vi "从板信息配置.vi"(2 "从板信息查看":string[][](table)) -> (0 "输出数组":string[][](array[string]), 1 "布尔":bool)   [LabVIEW 2013]
panel:
  in  "自动计算通道电压":bool
  in  "通道电压清零":bool
  in  "保险位置清零":bool
  in  "停止":bool
  in  "整车CAN测试":bool
  in  "保险位置":bool[][](array[boolean])
  in  "从板信息":string[][](table)=[["电压个数", "", "温度个数", "", "主板温度个数", "", "主板温度起始值"], ["电压起始值", "", "温度起始值", "", "从板1温度个数", "", "从板1主板温度起始值"]]
  in  "20个通道电压个数":u8[](array[numeric]) max=12
  # "1"
  # "2"
  # "3"
  # "4"
  # "5"
  # "6"
  # "7"
  # "8"
  # "9"
  # "10"
  # "11"
  # "12"
  # "第一通道"
  # "第二通道"
  # "第三通道"
  # "第四通道"
  # "第五通道"
  # "第六通道"
  # "第七通道"
  # "第八通道"
  # "第九通道"
  # "第十通道"
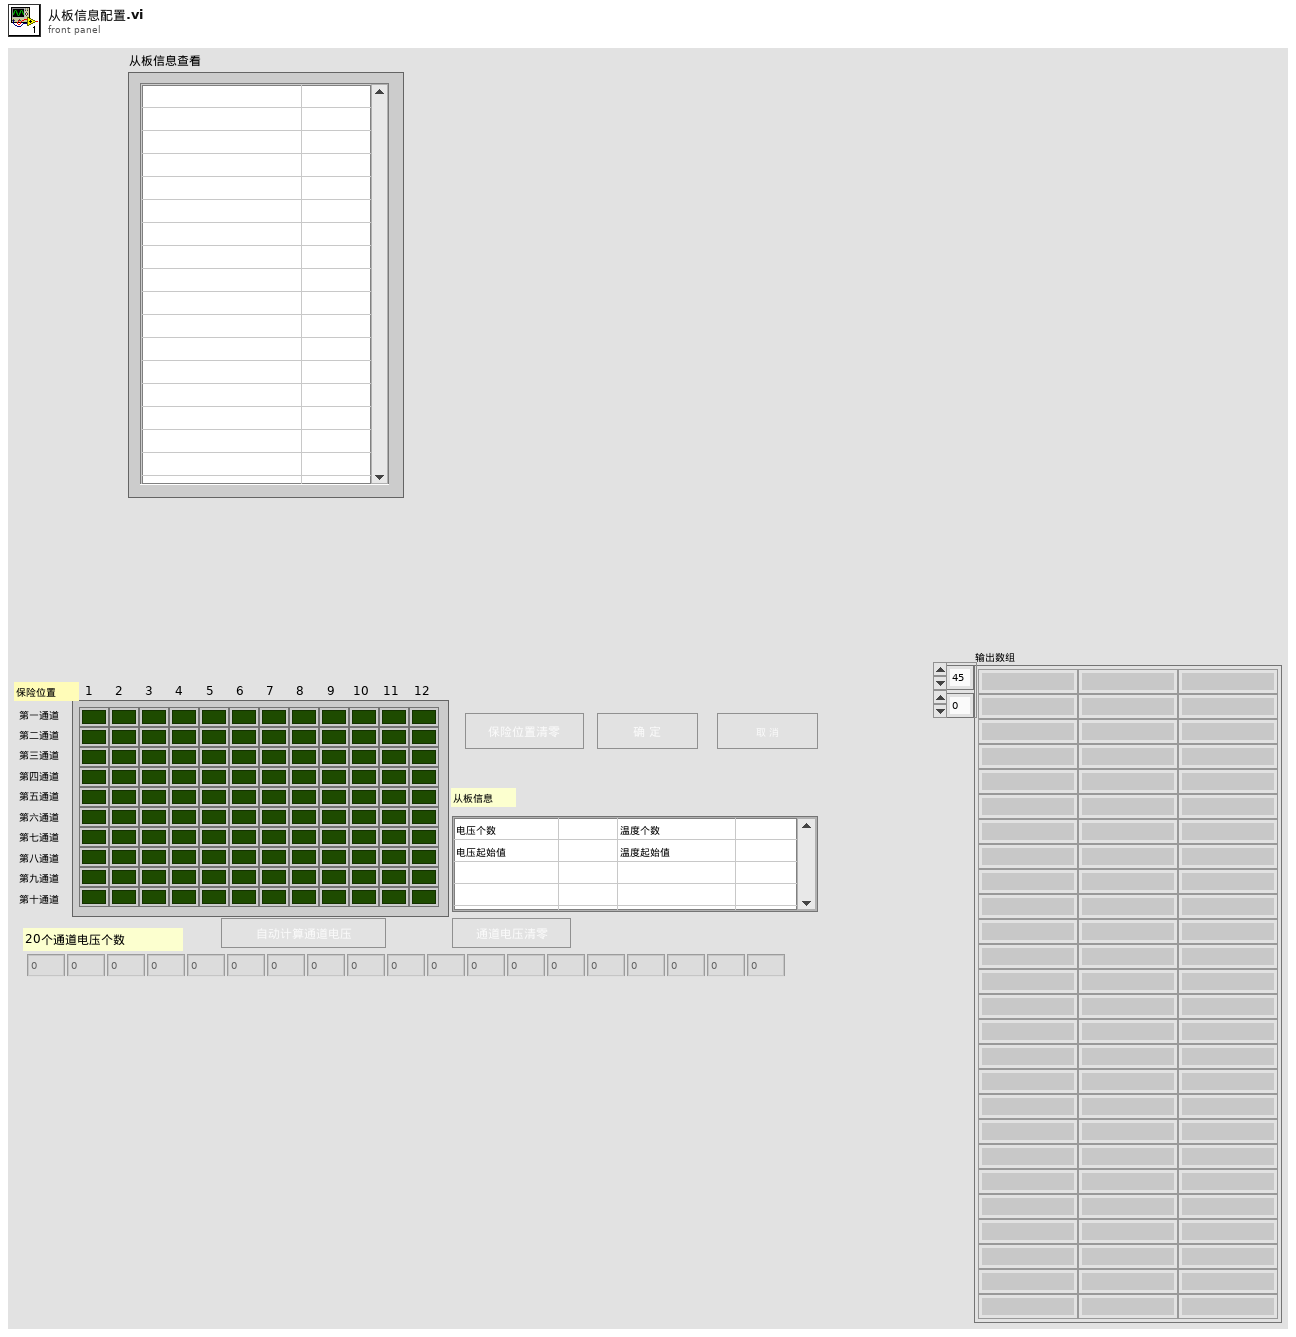
[diagram p1: front panel]
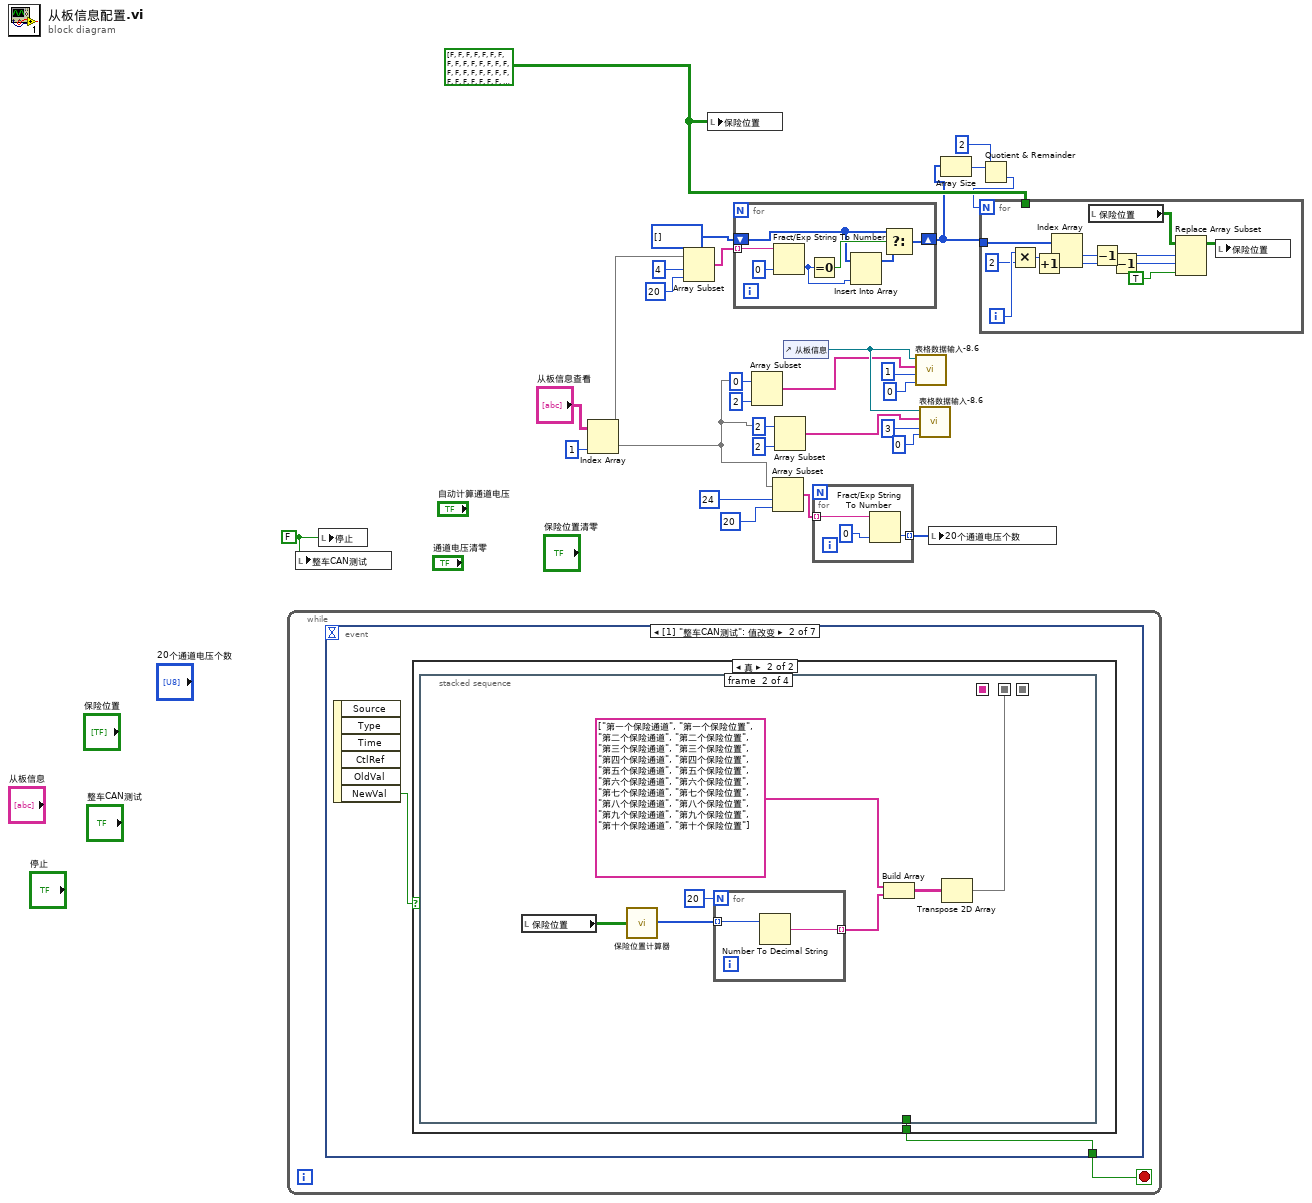
[diagram p0: block diagram]
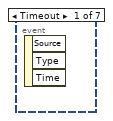
[diagram p2: hidden frame]
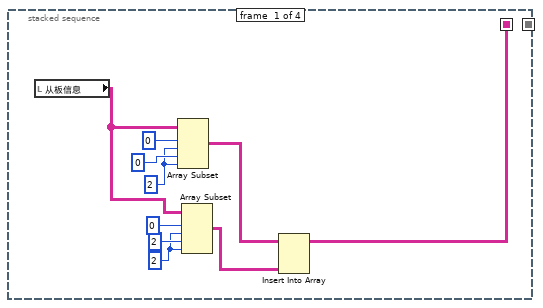
[diagram p4: hidden frame]
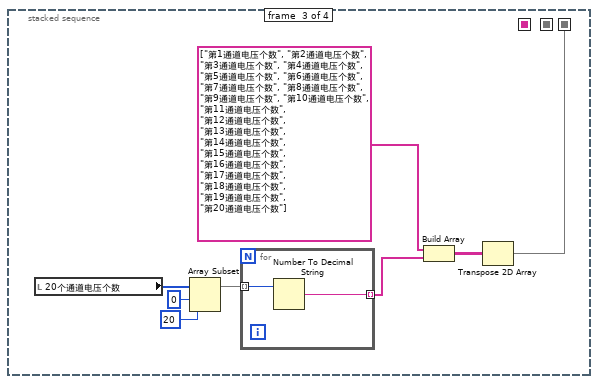
[diagram p5: hidden frame]
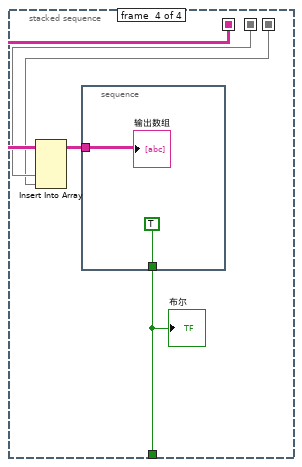
[diagram p6: hidden frame]
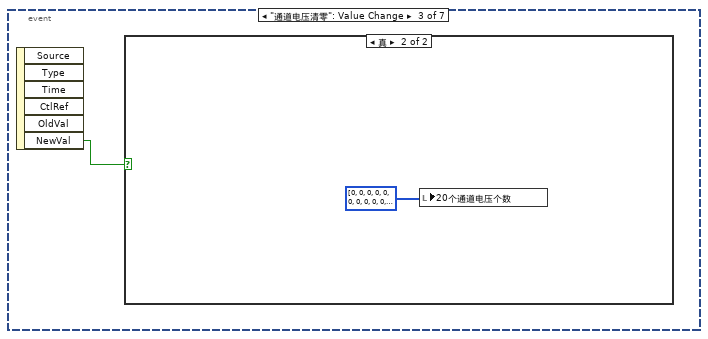
[diagram p7: hidden frame]
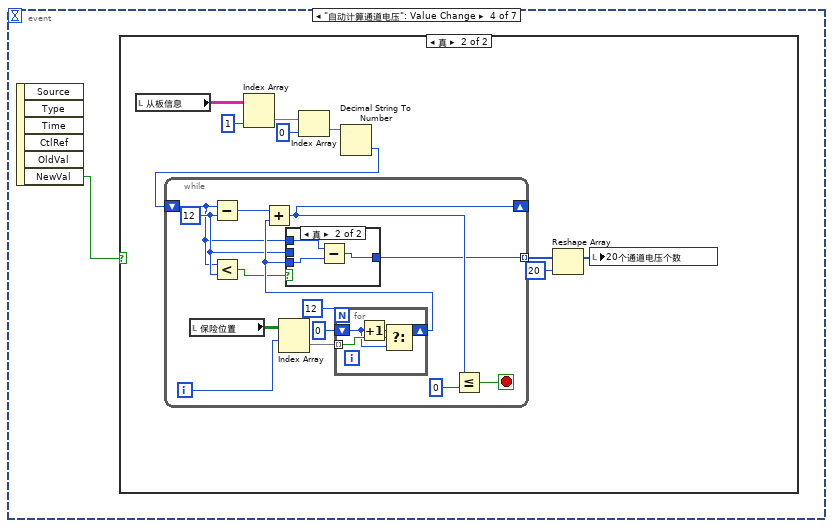
[diagram p9: hidden frame]
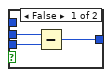
[diagram p11: hidden frame]
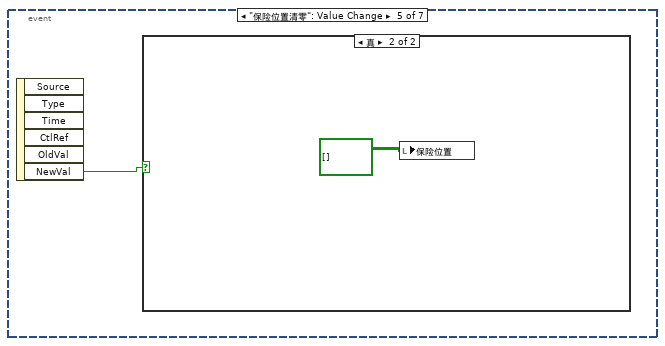
[diagram p12: hidden frame]
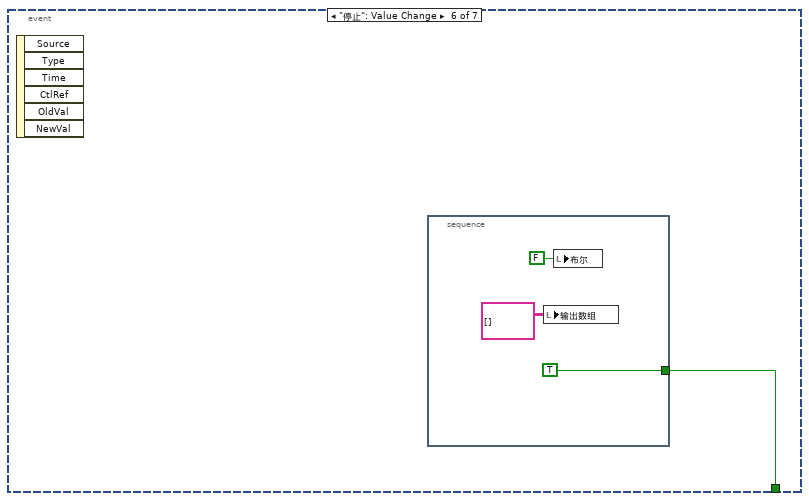
[diagram p14: hidden frame]
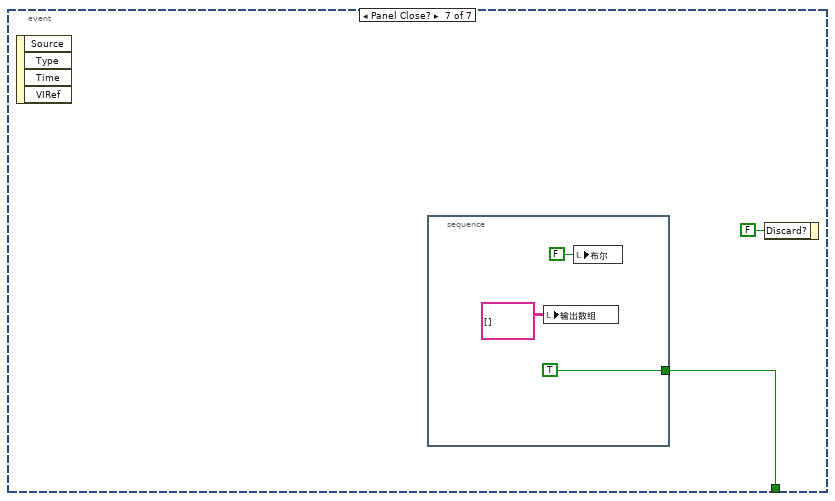
[diagram p15: hidden frame]
diagram:
  w6 = bool[][] [[FALSE, FALSE, FALSE, FALSE, FALSE, FALSE, FALSE, FALSE, FALSE, FALSE, FALSE, FALSE], [FALSE, FALSE, FALSE, FALSE, FALSE, FALSE, FALSE, FALSE, FALSE, FALSE, FALSE, FALSE], [FALSE, FALSE, FALSE, FALSE, FALSE, FALSE, FALSE, FALSE, FALSE, FALSE, FALSE, FALSE], [FALSE, FALSE, FALSE, FALSE, FALSE, FALSE, FALSE, FALSE, FALSE, FALSE, FALSE, FALSE], [FALSE, FALSE, FALSE, FALSE, FALSE, FALSE, FALSE, FALSE, FALSE, FALSE, FALSE, FALSE], [FALSE, FALSE, FALSE, FALSE, FALSE, FALSE, FALSE, FALSE, FALSE, FALSE, FALSE, FALSE], [FALSE, FALSE, FALSE, FALSE, FALSE, FALSE, FALSE, FALSE, FALSE, FALSE, FALSE, FALSE], [FALSE, FALSE, FALSE, FALSE, FALSE, FALSE, FALSE, FALSE, FALSE, FALSE, FALSE, FALSE], [FALSE, FALSE, FALSE, FALSE, FALSE, FALSE, FALSE, FALSE, FALSE, FALSE, FALSE, FALSE], [FALSE, FALSE, FALSE, FALSE, FALSE, FALSE, FALSE, FALSE, FALSE, FALSE, FALSE, FALSE]]
  w28 = FALSE ("取消按钮")
  n1 = while {
    stop <- w29 stop-if-true
    n2 = event shown="[1] \"整车CAN测试\": 值改变" {
      selector: _ -> [_ _ _ _ _ _ _]
      dyn-events: _ -> [_ _ _ _ _ _ _]
      timeout: _ -> [_ _ _ _ _ _ _]
      tunnel: [_ w30 _ _ _ w107 w112] -> w29
      event Timeout {
        n3 = event-data() -> ()  [unwired: 1 in, 3 out]
      }
      event "整车CAN测试": Value Change {
        n4 = event-data() -> ("NewVal"=w31:bool)  [unwired: 1 in, 5 out]
        n5 = case shown="真" w31 {
          tunnel: [_ w32] -> w30
          frame False {
          }
          frame True {
            n6 = stacked-sequence {
              seq-local: [w35 _ _ _] -> [_ _ _ w64]
              seq-local: [_ w44 _ _] -> [_ _ _ w63]
              seq-local: [_ _ w55 _] -> [_ _ _ w62]
              tunnel: [_ _ _ w65] -> w32
              frame #0 {
                w33 = 2 ("索引")
                w34 = 2 ("索引")
                n7 = local read "从板信息"() -> (w38:string[][])
                n8 = Array Subset(array=w38, index (row)=0 ("索引"), length (row)=w34, index (col)=0 ("索引"), length (col)=w34) -> (w37:string[][])
                n9 = Array Subset(array=w38, index (row)=0 ("索引"), length (row)=w33, index (col)=2 ("索引"), length (col)=w33) -> (w36:string[][])
                n10 = Insert Into Array(array=w37, new element=w36) -> (w35:string[][])  [unwired: 2 in]
              }
              frame #1 {
                n11 = local read "保险位置"() -> (w49:bool[][])
                n12 = call "保险位置计算器.vi"("保险位置"=w49) -> ("输出数组"=w48:i32[])
                n13 = for {
                  N: 20 -> [_]
                  tunnel: w48 -> [w51] mode=indexing
                  tunnel: [w50] -> w47 mode=indexing
                  n14 = Number To Decimal String(number=w51) -> (decimal integer string=w50:string)  [unwired: 1 in]
                }
                n15 = Build Array(string[] ["第一个保险通道", "第一个保险位置", "第二个保险通道", "第二个保险位置", "第三个保险通道", "第三个保险位置", "第四个保险通道", "第四个保险位置", "第五个保险通道", "第五个保险位置", "第六个保险通道", "第六个保险位置", "第七个保险通道", "第七个保险位置", "第八个保险通道", "第八个保险位置", "第九个保险通道", "第九个保险位置", "第十个保险通道", "第十个保险位置"], w47) -> (w45:string[][])
                n16 = Transpose 2D Array(2D array=w45) -> (transposed array=w44:string[][])
              }
              frame #2 {
                n17 = local read "20个通道电压个数"() -> (w59:u8[])
                n18 = Array Subset(array=w59, index=0 ("索引"), length=20 ("长度")) -> (w54:u8[])
                n19 = for {
                  tunnel: w54 -> [w61] mode=indexing
                  tunnel: [w60] -> w58 mode=indexing
                  n20 = Number To Decimal String(number=w61) -> (decimal integer string=w60:string)  [unwired: 1 in]
                }
                n21 = Build Array(string[] ["第1通道电压个数", "第2通道电压个数", "第3通道电压个数", "第4通道电压个数", "第5通道电压个数", "第6通道电压个数", "第7通道电压个数", "第8通道电压个数", "第9通道电压个数", "第10通道电压个数", "第11通道电压个数", "第12通道电压个数", "第13通道电压个数", "第14通道电压个数", "第15通道电压个数", "第16通道电压个数", "第17通道电压个数", "第18通道电压个数", "第19通道电压个数", "第20通道电压个数"], w58) -> (w56:string[][])
                n22 = Transpose 2D Array(2D array=w56) -> (transposed array=w55:string[][])
              }
              frame #3 {
                n23 = Insert Into Array(array=w64, new element #1=w63, new element #2=w62) -> (w66:string[][])  [unwired: 2 in]
                n24 = stacked-sequence {
                  tunnel: w66 -> [w68]
                  tunnel: [TRUE] -> w65
                  frame #0 {
                    "输出数组" <- w68
                  }
                }
                "布尔" <- w65
              }
            }
          }
        }
      }
      event "通道电压清零": Value Change {
        n25 = event-data() -> ("NewVal"=w69:bool)  [unwired: 1 in, 5 out]
        n26 = case shown="真" w69 {
          frame False {
          }
          frame True {
            n27 = local write "20个通道电压个数"(i32[] [0, 0, 0, 0, 0, 0, 0, 0, 0, 0, 0, 0, 0, 0, 0, 0, 0, 0, 0, 0, 0] ("20个通道电压个数")) -> ()
          }
        }
      }
      event "自动计算通道电压": Value Change {
        n28 = event-data() -> ("NewVal"=w71:bool)  [unwired: 1 in, 5 out]
        n29 = case shown="真" w71 {
          frame False {
          }
          frame True {
            n30 = local read "从板信息"() -> (w80:string[][])
            n31 = Index Array(array=w80, index (col)=1 ("禁用的索引 (列)")) -> (element=w78:string[])  [unwired: 1 in]
            n32 = Index Array(array=w78, index=0 ("索引")) -> (element=w76:string)
            n33 = Decimal String To Number(string=w76) -> (number=w75:i32)  [unwired: 2 in, 1 out]
            n34 = while {
              shift-right: [w86] -> _
              shift-left: w75 -> [w81]
              tunnel: [w84] -> w74 mode=indexing
              i -> [w93]
              stop <- w87 stop-if-true
              w83 = 12 ("y")
              n35 = local read "保险位置"() -> (w94:bool[][])
              n36 = Subtract(x=w81, y=w83) -> (x-y=w89:i32)
              n37 = Less?(x=w81, y=w83) -> (x < y?=w82:bool)
              n38 = Index Array(array=w94, index (row)=w93) -> (element=w92:bool[])  [unwired: 1 in]
              n39 = for {
                N: 12 -> [_]
                tunnel: w92 -> [w103] mode=indexing
                shift-right: [w104] -> w85
                shift-left: 0 -> [w101]
                n40 = Increment(x=w101) -> (x+1=w102:i32)
                n41 = Select(t=w102, s=w103, f=w101) -> (s? t:f=w104:i32)
              }
              n42 = Add(x=w89, y=w85) -> (x+y=w86:i32)
              n43 = case shown="真" w82 {
                tunnel: w85 -> [w97 w100]
                tunnel: [w96 w98] -> w84
                tunnel: w83 -> [w95 _]
                tunnel: w81 -> [_ w99]
                frame False {
                  n44 = Subtract(x=w95, y=w97) -> (x-y=w96:i32)
                }
                frame True {
                  n45 = Subtract(x=w99, y=w100) -> (x-y=w98:i32)
                }
              }
              n46 = Less Or Equal?(x=w86, y=0) -> (x <= y?=w87:bool)
            }
            n47 = Reshape Array(w74, 20 ("维数大小")) -> (w73:i32[])
            n48 = local write "20个通道电压个数"(w73) -> ()
          }
        }
      }
      event "保险位置清零": Value Change {
        n49 = event-data() -> ("NewVal"=w105:bool)  [unwired: 1 in, 5 out]
        n50 = case shown="真" w105 {
          frame False {
          }
          frame True {
            n51 = local write "保险位置"(bool[][] []) -> ()
          }
        }
      }
      event "停止": Value Change {
        n52 = event-data() -> ()  [unwired: 1 in, 6 out]
        n53 = stacked-sequence {
          tunnel: [TRUE] -> w107
          frame #0 {
            n54 = local write "输出数组"(string[][] [] ("输出数组")) -> ()
            n55 = local write "布尔"(FALSE ("布尔")) -> ()
          }
        }
      }
      event Panel Close? {
        n56 = event-data() -> ()  [unwired: 1 in, 4 out]
        n57 = stacked-sequence {
          tunnel: [TRUE] -> w112
          frame #0 {
            n58 = local write "输出数组"(string[][] [] ("输出数组")) -> ()
            n59 = local write "布尔"(FALSE ("布尔")) -> ()
          }
        }
        n60 = event-data("Discard?"=FALSE ("放弃？")) -> ()  [unwired: 1 in, 1 out]
      }
    }
  }
  n61 = local write "整车CAN测试"(w28) -> ()
  n62 = local write "停止"(w28) -> ()
  n63 = Index Array(array="从板信息查看", index (col)=1 ("禁用的索引 (列)")) -> (element=w8:string[])  [unwired: 1 in]
  n64 = Array Subset(array=w8, index=4 ("索引"), length=20 ("长度")) -> (w7:string[])
  n65 = local write "保险位置"(w6) -> ()
  n66 = for {
    tunnel: w7 -> [w122] mode=indexing
    shift-right: [w119] -> w4
    shift-left: i32[] [] -> [w118]
    n67 = Fract/Exp String To Number(string=w122, default (0 dbl)=u8 0) -> (number=w117:u8)  [unwired: 2 in, 1 out]
    n68 = Equal To 0?(x=w117) -> (x = 0?=w120:bool)
    n69 = Insert Into Array(array=w118, new element=w117) -> (w116:i32[])  [unwired: 1 in]
    n70 = Select(t=w118, s=w120, f=w116) -> (s? t:f=w119:i32[])
  }
  n71 = Array Subset(array=w8, index=0 ("索引"), length=2 ("长度")) -> (w14:string[])
  n72 = Array Subset(array=w8, index=24 ("索引"), length=20 ("长度")) -> (w12:string[])
  n73 = Array Subset(array=w8, index=2 ("索引"), length=2 ("长度")) -> (w13:string[])
  n74 = control-ref of="从板信息"() -> (w16:refnum<vi>)
  n75 = for {
    tunnel: w12 -> [w125] mode=indexing
    tunnel: [w124] -> w11 mode=indexing
    n76 = Fract/Exp String To Number(string=w125, default (0 dbl)=u8 0) -> (number=w124:u8)  [unwired: 2 in, 1 out]
  }
  n77 = call "表格数据输入-8.6.vi"("行数"=u32 0, "列数"=u32 1 ("行数"), "字符串数组"=w14, "表格引用"=w16) -> ()  [unwired: 8 in]
  n78 = call "表格数据输入-8.6.vi"("行数"=u32 0, "列数"=u32 3 ("行数"), "字符串数组"=w13, "表格引用"=w16) -> ()  [unwired: 8 in]
  n79 = local write "20个通道电压个数"(w11) -> ()
  n80 = Array Size(array=w4) -> (size(s)=w3:i32)
  n81 = Quotient & Remainder(x=w3, y=2) -> (floor(x/y)=w1:i32)  [unwired: 1 out]
  n82 = for {
    N: w1 -> [_]
    tunnel: w4 -> [w137]
    tunnel: w6 -> [_]
    i -> [w136]
    n83 = Multiply(x=w136, y=2) -> (x*y=w134:i32)
    n84 = Increment(x=w134) -> (x+1=w133:i32)
    n85 = Index Array(array=w137, index #1=w134, index #2=w133) -> (element #1=w132:i32, element #2=w129:i32)
    n86 = local read "保险位置"() -> (w130:bool[][])
    n87 = Decrement(x=w132) -> (x-1=w127:i32)
    n88 = Decrement(x=w129) -> (x-1=w126:i32)
    n89 = Replace Array Subset(array=w130, new element=TRUE, index (row)=w127, index (col)=w126) -> (w131:bool[][])
    n90 = local write "保险位置"(w131) -> ()
  }
